vi "PM100D_GetRngLbl.vi"(0 "PM100D":refnum<visa-resource-name>, 1 "MainUnits":enum16{"W", "V", "J", "dBm", "A"}(ring)) -> (2 "String":string, 3 "Numeric":dbl, 4 "Auto":bool)   [LabVIEW 2015]
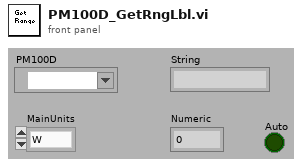
[diagram p1: front panel]
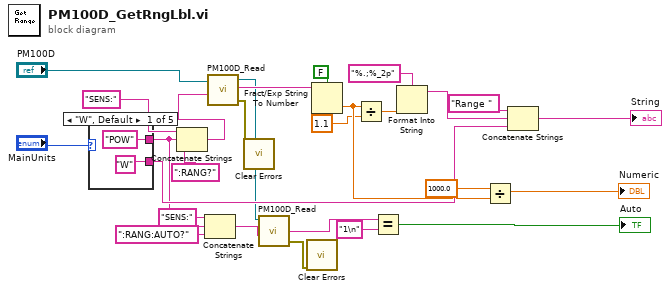
[diagram p0: block diagram]
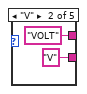
[diagram p2: hidden frame]
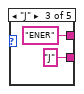
[diagram p3: hidden frame]
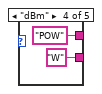
[diagram p4: hidden frame]
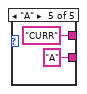
[diagram p5: hidden frame]
diagram:
  n1 = case shown="\"W\", Default" "MainUnits" {
    tunnel: ["POW" "VOLT" "ENER" "POW" "CURR"] -> w8
    tunnel: ["W" "V" "J" "W" "A"] -> w25
    frame "W", Default {
    }
    frame "V" {
    }
    frame "J" {
    }
    frame "dBm" {
    }
    frame "A" {
    }
  }
  n2 = Concatenate Strings("SENS:" ("string"), w8, ":RANG?" ("string")) -> (w23:string)
  n3 = Concatenate Strings("SENS:" ("string"), w8, ":RANG:AUTO?" ("string")) -> (w6:string)
  n4 = call "PM100D_Read.vi"("Command"=w23, "VISA in"="PM100D") -> ("error out"=w11:errorcluster, "ReadValue"=w16:string, "VISA out"=w10:refnum<visa-resource-name>)  [unwired: 2 in]
  n5 = call <vilib>:"Clear Errors.vi"("error in (no error)"=w11) -> ()  [unwired: 5 in, 2 out]
  n6 = call "PM100D_Read.vi"("Command"=w6, "VISA in"=w10) -> ("error out"=w9:errorcluster, "ReadValue"=w5:string)  [unwired: 2 in, 1 out]
  n7 = call <vilib>:"Clear Errors.vi"("error in (no error)"=w9) -> ()  [unwired: 5 in, 2 out]
  n8 = Fract/Exp String To Number(use system decimal point (T)=FALSE, string=w16) -> (number=w21:dbl)  [unwired: 2 in, 1 out]
  n9 = Divide(x=w21, y=1.1) -> (x/y=w13:dbl)
  n10 = Equal?(x=w5, y="1\n") -> (x = y?=→"Auto":bool)
  n11 = Format Into String(format string="%.;%_2p", w13) -> (resulting string=w26:string)  [unwired: 2 in, 1 out]
  n12 = Divide(x=1000.0, y=w21) -> (x/y=→"Numeric":dbl)
  n13 = Concatenate Strings("Range " ("string"), w26, w25) -> (→"String":string)
